vi "Calculate_travel_time.vi"(1 "Default Acceleration":dbl format="%.2f", 2 "Default Velocity":dbl format="%.2f", 3 "Revs to travel":dbl format="%.4f") -> (0 "Times":T1 {"Accelation fractional distance" format="%.2f"; "Accelaration time" format="%.7f"; "Total travel time" format="%.7f"})   [LabVIEW 2010]
panel:
  out "Revs to Accel to V":dbl format="%.2f"
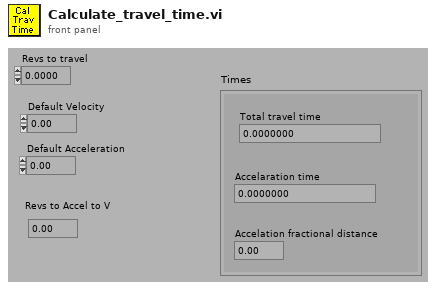
[diagram p1: front panel]
types:
  T1 = cluster{"Total travel time":dbl, "Accelaration time":dbl, "Accelation fractional distance":dbl}
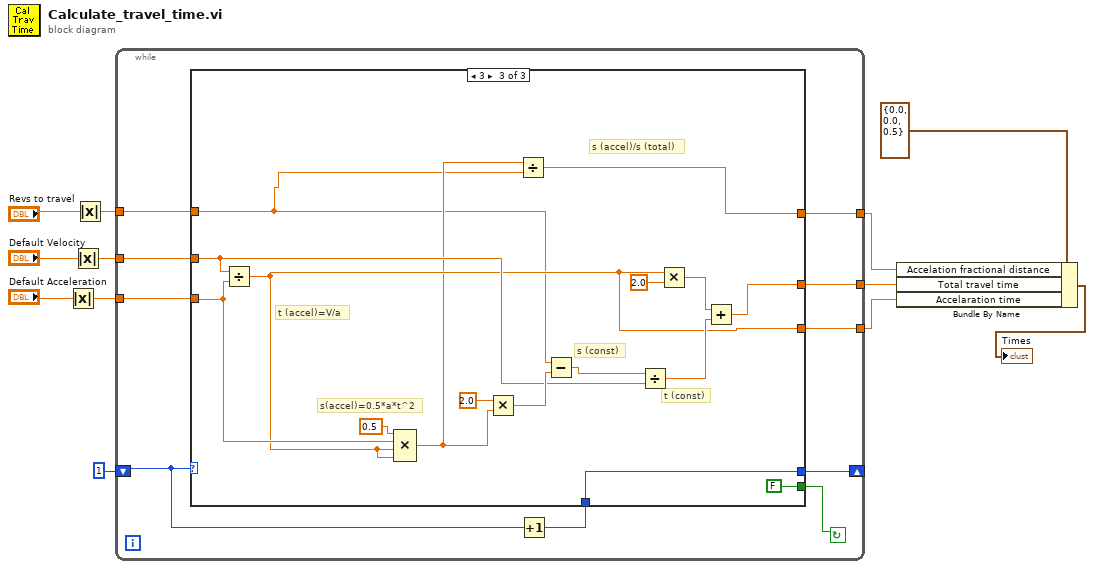
[diagram p0: block diagram]
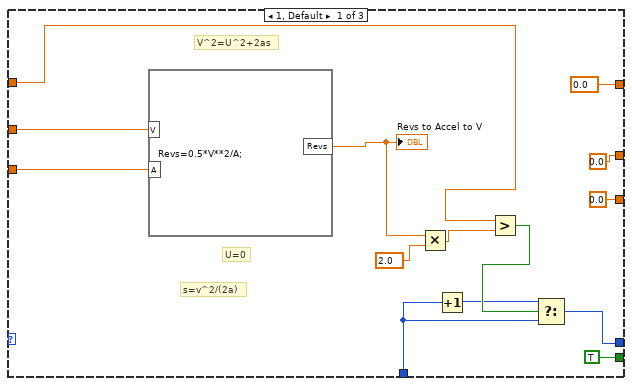
[diagram p2: hidden frame]
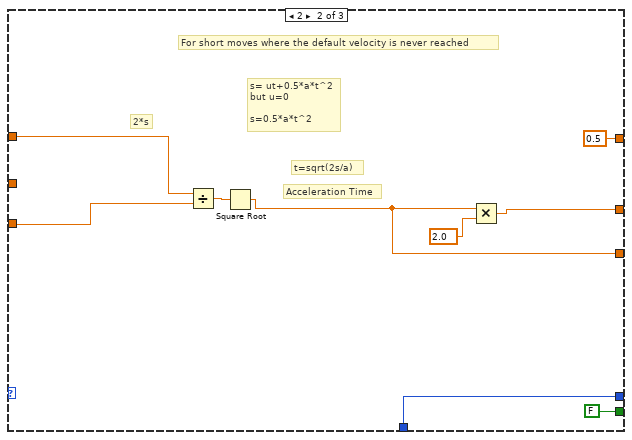
[diagram p3: hidden frame]
diagram:
  n1 = Absolute Value(x="Default Acceleration") -> (abs(x)=w6:dbl)
  n2 = Absolute Value(x="Default Velocity") -> (abs(x)=w7:dbl)
  n3 = Absolute Value(x="Revs to travel") -> (abs(x)=w8:dbl)
  n4 = while {
    tunnel: w8 -> [w16]
    tunnel: w6 -> [w17]
    tunnel: w7 -> [w18]
    shift-left: 1 -> [w22]
    shift-right: [w20] -> _
    tunnel: [w15] -> w2
    tunnel: [w14] -> w1
    tunnel: [w13] -> w3
    stop <- w19 continue-if-true
    n5 = Increment(x=w22) -> (x+1=w21:i32)
    n6 = case shown="3" w22 {
      tunnel: w21 -> [w31 w43 w61]
      tunnel: [w29 w43 w61] -> w20
      tunnel: [TRUE FALSE FALSE] -> w19
      tunnel: w18 -> [w28 _ w54]
      tunnel: w17 -> [w27 w40 w58]
      tunnel: w16 -> [w26 w41 w46]
      tunnel: [0.0 w39 w50] -> w15
      tunnel: [0.0 w38 w49] -> w14
      tunnel: [0.0 ("y") 0.5 ("y") w48] -> w13
      frame 1, Default {
        # "s=v^2/(2a)"
        # "U=0"
        # "V^2=U^2+2as"
        n7 = formula code="Revs=0.5*V**2/A;"("V"=w28, "A"=w27) -> ("Revs"=w36:dbl)
        "Revs to Accel to V" <- w36
        n8 = Multiply(x=w36, y=2.0) -> (x*y=w34:dbl)
        n9 = Increment(x=w31) -> (x+1=w30:i32)
        n10 = Greater?(x=w26, y=w34) -> (0:w32:bool)
        n11 = Select(t=w30, s=w32, f=w31) -> (s? t:f=w29:i32)
      }
      frame 2 {
        # "s= ut+0.5*a*t^2\nbut u=0\n\ns=0.5*a*t^2"
        # "t=sqrt(2s/a)"
        # "2*s"
        # "For short moves where the default velocity is never reached"
        # "Acceleration Time"
        n12 = Divide(x=w41, y=w40) -> (x/y=w45:dbl)
        n13 = Square Root(x=w45) -> (sqrt(x)=w38:dbl)
        n14 = Multiply(x=w38, y=2.0) -> (x*y=w39:dbl)
      }
      frame 3 {
        # "s (accel)/s (total)"
        # "t (const)"
        # "s (const)"
        # "s(accel)=0.5*a*t^2"
        # "t (accel)=V/a"
        n15 = Divide(x=w54, y=w58) -> (x/y=w49:dbl)
        n16 = Compound Arithmetic op=MULTIPLY(0.5 ("y"), w58, w49, w49) -> (w47:dbl)
        n17 = Multiply(x=2.0, y=w47) -> (x*y=w56:dbl)
        n18 = Divide(x=w47, y=w46) -> (x/y=w48:dbl)
        n19 = Subtract(x=w46, y=w56) -> (x-y=w55:dbl)
        n20 = Divide(x=w55, y=w54) -> (x/y=w52:dbl)
        n21 = Multiply(x=w49, y=2.0) -> (x*y=w51:dbl)
        n22 = Add(x=w51, y=w52) -> (x+y=w50:dbl)
      }
    }
  }
  n23 = Bundle By Name(cluster=T1 {"Total travel time"=0.0, "Accelaration time"=0.0, "Accelation fractional distance"=0.5} ("Times"), "Accelation fractional distance"=w3, "Total travel time"=w2, "Accelaration time"=w1) -> (→"Times":T1)
